vi "PlotSS.vi"(0 "X-Axis Array (nm) In":dbl[][](array[numeric]), 1 "Mode":T7, 2 "StoreInto":u16(ring) items=["Store Into", "Previous", "older", "Ref#1", "Ref#2", "Ref#3", "Ref#4", "Ref#5", "Ref#6", "Ref#7"], 3 "Fixed items":bool[](array[boolean]), 5 "X-Axis":i32, 7 "Data Array In":dbl[][](array[numeric]), 9 "Print":bool, 11 "File Info Buffer Input":T1[](array[typedef]) {"CCD Parameters"."dt or s" format="%#.6f"; "CCD Parameters"."Repetition" min=1; "CCD Parameters"."Offset" format="%#.2f"; "CCD Parameters"."Exposure Time (s)" min=0.02 max=6000.0 format="%#.2f"; "Center nm" format="%.2f"; "Temperature (K)" format="%.2f"; "Field (T)" format="%.2f"}, 12 "Show/hide":bool[](array[boolean]), 13 "Data Plot Input":cluster{dbl[], dbl[]}[](graph)) -> (4 "X-Axis Array (nm) Out":dbl[][](array[numeric]), 8 "Data Array Out":dbl[][](array[numeric]), 14 "Data Plot":cluster{dbl[], dbl[]}[](graph), 15 "File Info Buffer Out":T1[](array[typedef]) {"CCD Parameters"."dt or s" format="%#.6f"; "CCD Parameters"."Repetition" min=1; "CCD Parameters"."Offset" format="%#.2f"; "CCD Parameters"."Exposure Time (s)" min=0.02 max=6000.0 format="%#.2f"; "Center nm" format="%.2f"; "Temperature (K)" format="%.2f"; "Field (T)" format="%.2f"})   [LabVIEW 2019]
uses:
  PlottSS.ctl
  Globals and TypeDefs/Type Definitions.llb/FileInfoParameter.ctt
  Globals and TypeDefs/Type Definitions.llb/Wavelength Unit.ctt
  Globals and TypeDefs/Type Definitions.llb/McPherson Grating Density.ctl
  Globals and TypeDefs/Type Definitions.llb/CCDParameter.ctt
  Globals and TypeDefs/Type Definitions.llb/OperationMode.ctt
  Globals and TypeDefs/Type Definitions.llb/ListOfDetectors.ctt
  Sub VIs/File and save/X-Axis Converter.llb/X-Axis Converter.vi
panel:
  in  "Most recent saved file":path=path "erererere"
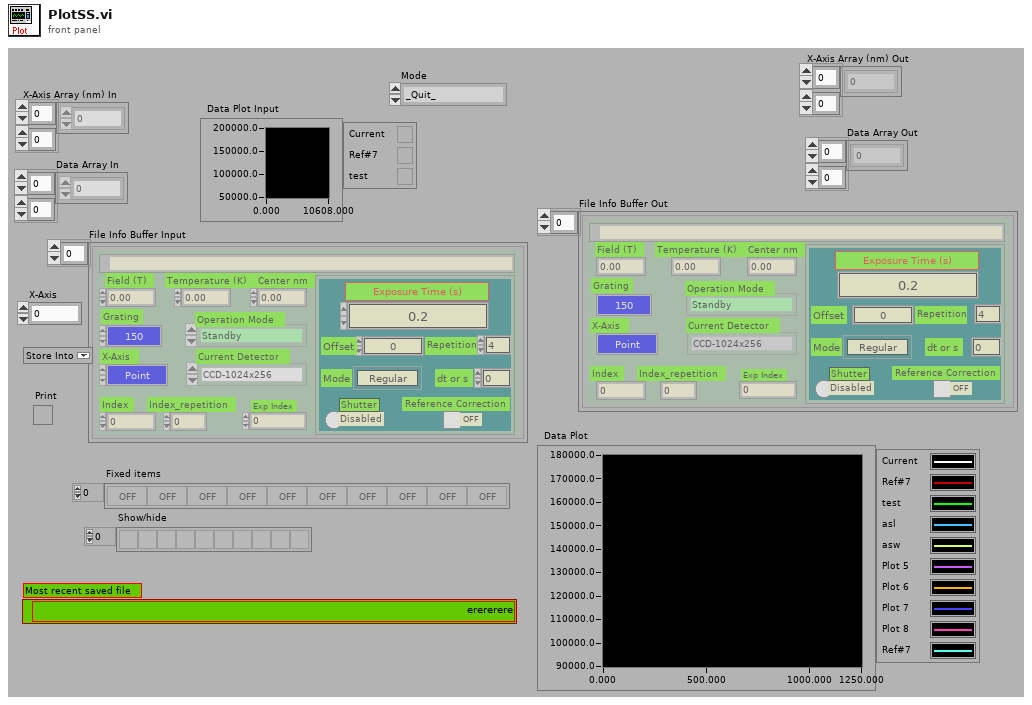
[diagram p1: front panel]
types:
  T1 = typedef "FileInfoParameter.ctt" = cluster{"FilePath":path, "Field (T)":dbl, "Temperature (K)":dbl, "X-Axis":T2, "Center nm":dbl, "Current Grating Density":T3, "CCD Parameters":T4, "Operation Mode":T5, "Exp Index":u32, "Index_repetition":u16, "Index":u16, "Current Detector":T6}
  T2 = typedef "Wavelength Unit.ctt" = enum8{"Point", "nm", "eV", "meV", "cm_1"}
  T3 = typedef "McPherson Grating Density.ctl" = enum8{"150", "300", "600", "1200", "1800"}
  T4 = typedef "CCDParameter.ctt" = cluster{"Exposure Time (s)":dbl, "Offset":dbl, "BkgrdCrct":bool, "Shutter":bool, "Mode":enum8{"Regular", "OverExp Cor", "SpikeRemove", "ForCalibration"}, "Repetition":u16, "dt or s":dbl}
  T5 = typedef "OperationMode.ctt" = enum16{"Standby", "CCD Single Shot", "CCD Sequence Shots", "CCD Custom Shots", "CCD Reference Shot", "Step Scanning ", "Time Scanning", "NML Data Acquisition"}
  T6 = typedef "ListOfDetectors.ctt" = enum8{"CCD-1024x256", "InGaAs PDA-1024x1", "CCD-1340x400", "Ge Single Channel", "Si Single Channel", "PMT Single Channel"}
  T7 = typedef "PlottSS.ctl" = enum16{"_Quit_", "Init", "load", "Pin-Mix", "Trace-Show/Hide", "Unit-Change", "Display/Print", "Column Heading"}
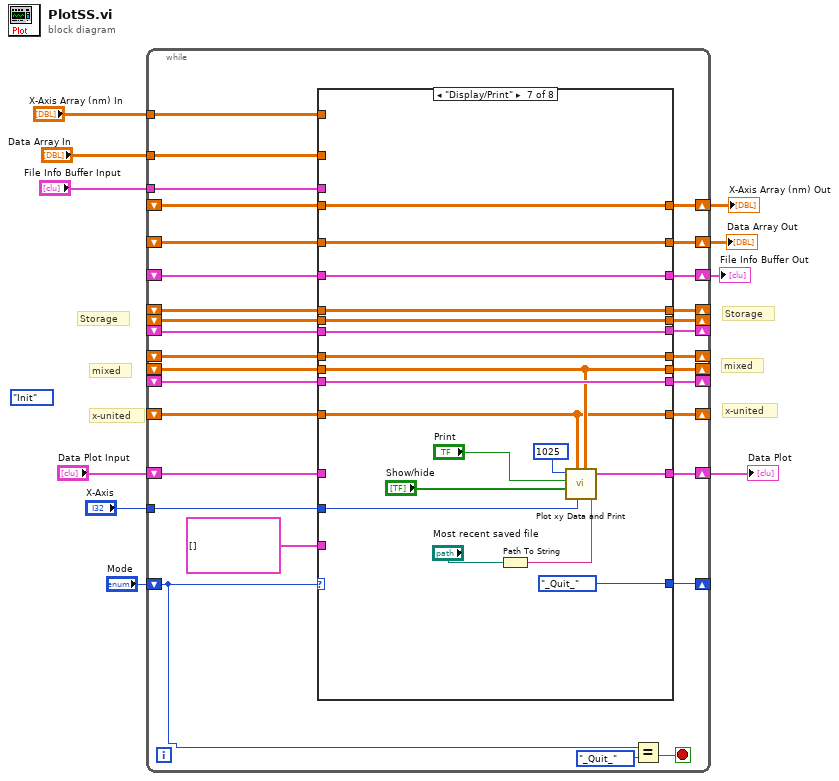
[diagram p0: block diagram]
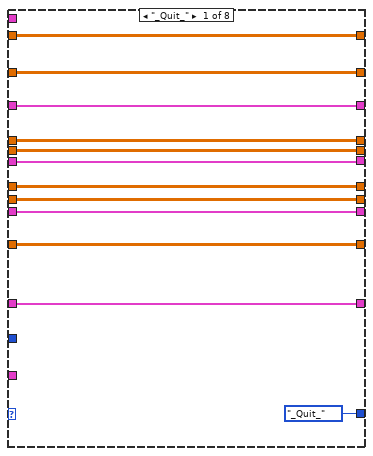
[diagram p2: hidden frame]
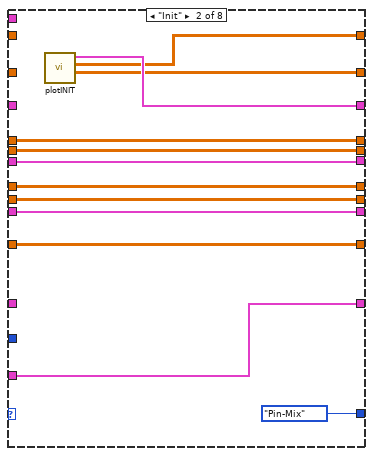
[diagram p3: hidden frame]
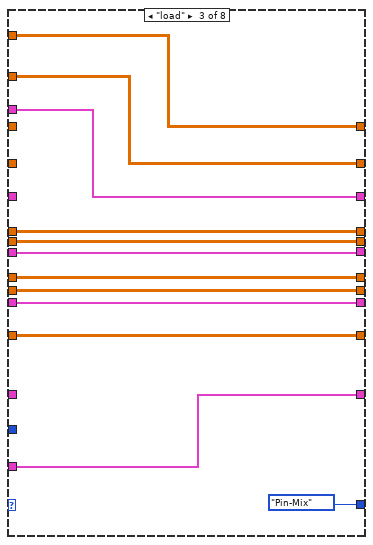
[diagram p4: hidden frame]
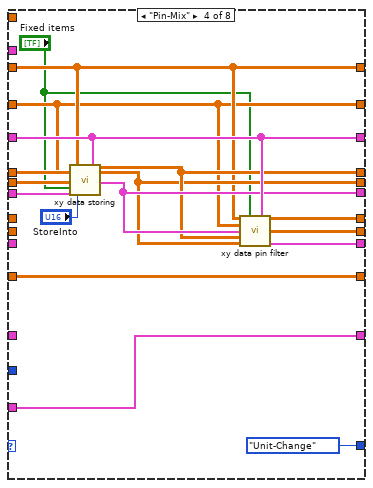
[diagram p5: hidden frame]
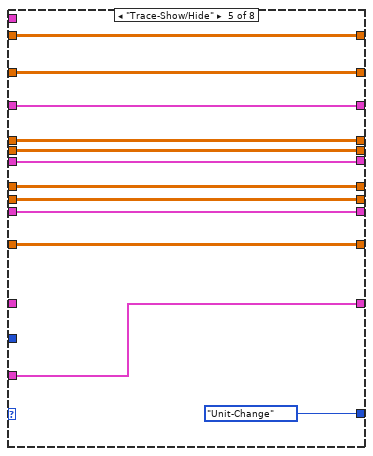
[diagram p6: hidden frame]
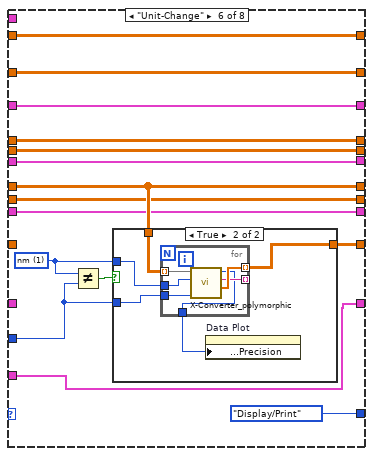
[diagram p7: hidden frame]
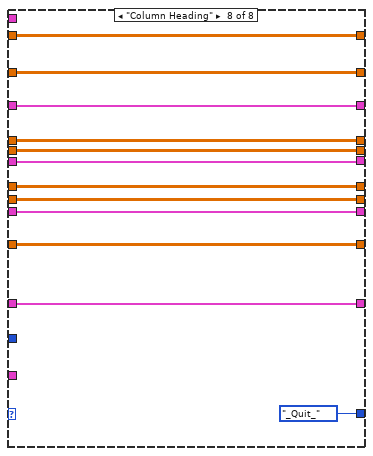
[diagram p9: hidden frame]
diagram:
  (unwired) PlottSS."Init"
  # "x-united"
  # "mixed"
  # "Storage"
  # "x-united"
  # "mixed"
  # "Storage"
  n1 = while {
    shift-right: [w40] -> _
    shift-left: "Mode" -> [w41]
    shift-right: [w35] -> w9
    shift-left: _ -> [w37]
    shift-right: [w34] -> w8
    shift-left: _ -> [w36]
    shift-right: [w32] -> w6
    shift-left: _ -> [w33]
    shift-right: [w30] -> _
    shift-left: _ -> [w31]
    shift-right: [w27] -> _
    shift-left: _ -> [w29]
    shift-right: [w26] -> _
    shift-left: _ -> [w28]
    shift-right: [w25] -> _
    shift-left: _ -> [w19]
    shift-right: [w24] -> _
    shift-left: _ -> [w22]
    shift-right: [w23] -> _
    shift-left: _ -> [w20]
    shift-right: [w21] -> _
    shift-left: _ -> [w18]
    tunnel: "X-Axis" -> [w17]
    tunnel: "X-Axis Array (nm) In" -> [w16]
    tunnel: "Data Array In" -> [w15]
    tunnel: "File Info Buffer Input" -> [w14]
    shift-right: [w13] -> w2
    shift-left: "Data Plot Input" -> [w12]
    stop <- w39 stop-if-true
    n2 = case shown="\"Display/Print\"" w41 {
      tunnel: [PlottSS."_Quit_" PlottSS."Pin-Mix" PlottSS."Pin-Mix" PlottSS."Unit-Change" PlottSS."Unit-Change" PlottSS."Display/Print" PlottSS."_Quit_" PlottSS."_Quit_"] -> w40
      tunnel: [w52 w63 w69 w82 w105 w117 w150 w162] -> w35
      tunnel: w37 -> [w52 _ _ w82 w105 w117 w150 w162]
      tunnel: [w51 w62 w68 w81 w104 w116 w149 w161] -> w34
      tunnel: w36 -> [w51 _ _ w81 w104 w116 w149 w161]
      tunnel: [w50 w64 w67 w91 w103 w115 w148 w160] -> w32
      tunnel: w33 -> [w50 _ _ w91 w103 w115 w148 w160]
      tunnel: w31 -> [w47 w59 w74 w84 w100 w112 w145 w157]
      tunnel: [w47 w59 w74 w90 w100 w112 w145 w157] -> w30
      tunnel: w29 -> [w49 w61 w76 w93 w102 w114 w147 w159]
      tunnel: w28 -> [w48 w60 w75 w92 w101 w113 w146 w158]
      tunnel: [w49 w61 w76 w89 w102 w114 w147 w159] -> w27
      tunnel: [w48 w60 w75 w88 w101 w113 w146 w158] -> w26
      tunnel: [w44 w56 w71 w87 w97 w109 w143 w154] -> w25
      tunnel: [w46 w58 w73 w86 w99 w111 w144 w156] -> w24
      tunnel: [w45 w57 w72 w85 w98 w110 w139 w155] -> w23
      tunnel: w22 -> [w46 w58 w73 _ w99 w111 w144 w156]
      tunnel: [w43 w55 w70 w80 w96 w118 w134 w153] -> w21
      tunnel: w20 -> [w45 w57 w72 _ w98 w110 w139 w155]
      tunnel: w19 -> [w44 w56 w71 _ w97 w109 w143 w154]
      tunnel: w18 -> [w43 w55 w70 w80 w96 _ w134 w153]
      tunnel: w17 -> [_ _ _ _ _ w108 w136 _]
      tunnel: w16 -> [_ _ w69 _ _ _ _ _]
      tunnel: w15 -> [_ _ w68 _ _ _ _ _]
      tunnel: w14 -> [_ _ w67 _ _ _ _ _]
      tunnel: [w42 w54 w66 w78 w95 w107 w135 w152] -> w13
      tunnel: w12 -> [w42 _ _ _ _ _ _ w152]
      tunnel: cluster{dbl[], dbl[]}[] [] -> [_ w54 w66 w78 w95 w107 _ _]
      frame "_Quit_" {
      }
      frame "Init" {
        n3 = call "plotINIT.vi"() -> ("Data Array output"=w62:dbl[][], "X-Axis Array output"=w63:dbl[][], "File Info Buffer Out"=w64:T1[])  [unwired: 1 in, 2 out]
      }
      frame "load" {
      }
      frame "Pin-Mix" {
        n4 = call "xy data storing.vi"("X-ArrayStorage Input"=w93, "Y-ArrayStorage Input"=w92, "Pinning Input"="Fixed items", "File Info Storage Input"=w84, "xData Input"=w82, "StoreInto"="StoreInto", "yData Input"=w81, "File Info Input"=w91) -> ("X-ArrayStorage Output"=w89:dbl[][], "Y-ArrayStorage Output"=w88:dbl[][], "File Info Storage Output"=w90:T1[])  [unwired: 4 in, 5 out]
        n5 = call "xy data pin filter.vi"("X-Axis Array Input"=w82, "Fixed items"="Fixed items", "File Info Input"=w91, "Data Array Input"=w81, "File Info Old"=w90, "X-Axis Array Old"=w89, "Data Array Old"=w88) -> ("X-Axis Array output"=w86:dbl[][], "Data Array output"=w85:dbl[][], "File Info Output"=w87:T1[])  [unwired: 6 in]
      }
      frame "Trace-Show/Hide" {
      }
      frame "Unit-Change" {
        w119 = 1 items=["Point #", "nm", "eV", "meV", "cm-1"] ("Old X-Axis Unit")
        n6 = Not Equal?(x=w119, y=w108) -> (x != y?=w120:bool)
        n7 = case shown="True" w120 {
          tunnel: w108 -> [_ w126]
          tunnel: [w122 w127] -> w118
          tunnel: w111 -> [w122 w125]
          tunnel: w119 -> [_ w124]
          frame False {
          }
          frame True {
            n8 = for {
              tunnel: [w133] -> w127 mode=indexing
              tunnel: w126 -> [w132]
              tunnel: [w131] -> _ mode=indexing
              tunnel: w125 -> [w130] mode=indexing
              tunnel: w124 -> [w129]
              tunnel: [w128] -> w123
              n9 = call-poly "X-Converter_polymorphic.vi"("X-Axis Unit"=w132, "Old X-Axis Unit"=w129, "X-Axis input"=w130) -> ("X-Axis Output"=w133:dbl[], "X-Axis Unit String"=w131:string, "Precision"=w128:i32)  [unwired: 2 in, 1 out]
            }
            n10 = property on="Data Plot" class="XYGraph (strict)"("X Scale.Format & Precision:Precision"=w123) -> ()  [unwired: 2 in, 2 out]
          }
        }
      }
      frame "Display/Print" {
        n11 = Path To String(path="Most recent saved file") -> (string=w141:string)
        n12 = call "Plot xy Data and Print.vi"("File:"=w141, "Data"=w139, "x axis column"=w136, "Display/hide"="Show/hide", "X-Axis Data"=w134, "Print"="Print", "Index"=1025) -> ("Data Plot"=w135:cluster{dbl[], dbl[]}[])  [unwired: 2 in, 1 out]
      }
      frame "Column Heading" {
      }
    }
    n13 = Equal?(x=w41, y=PlottSS."_Quit_") -> (x = y?=w39:bool)
  }
  "X-Axis Array (nm) Out" <- w9
  "Data Array Out" <- w8
  "File Info Buffer Out" <- w6
  "Data Plot" <- w2
